vi "Get SMO Public API.vi"(8 "error in (no error)":errorcluster, 11 "Sequence Experiment":refnum<class "Control Experiment.lvclass">) -> (0 "error out":errorcluster, 2 "Commands":string[](array[string]), 3 "Sequence Experiment out":refnum<class "Control Experiment.lvclass">)   [LabVIEW 2016, in "Control Experiment.lvclass"]
uses:
  Control Experiment.lvclass
  <userlib>/LevyLab/Levylab Instruments/SMOs/Instrument/Instrument.lvclass
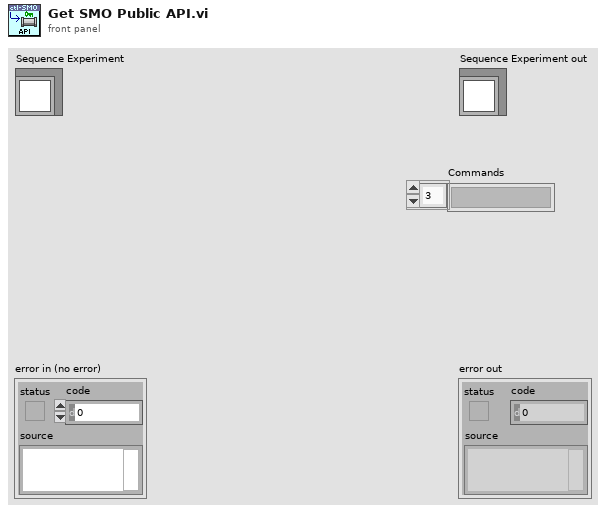
[diagram p1: front panel]
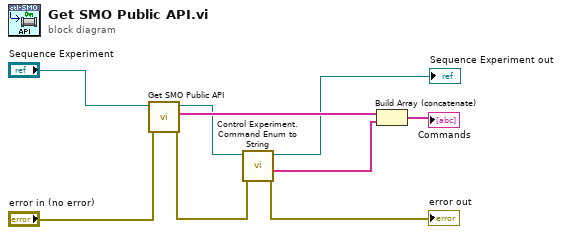
[diagram p0: block diagram]
diagram:
  n1 = call-parent "Get SMO Public API.vi"("error in (no error)"="error in (no error)", "Instrument in"="Sequence Experiment") -> ("error out"=w5:errorcluster, "Commands"=w9:string[], "Instrument out"=w3:refnum<class "Control Experiment.lvclass">)  [unwired: 7 in]
  n2 = call "Control Experiment.Command Enum to String.vi"("error in (no error)"=w5, "Sequence Experiment"=w3) -> ("error out"=→"error out":errorcluster, "Commands []"=w1:string[], "Sequence Experiment out"=→"Sequence Experiment out":refnum<class "Control Experiment.lvclass">)  [unwired: 6 in, 1 out]
  n3 = Build Array (concatenate)(w9, w1) -> (→"Commands":string[])
